vi "Demo.vi"() -> ()   [LabVIEW 2012, in "ProcessClass.lvclass"]
uses:
  ProcessClass.lvclass
panel:
  out "Process Names":string[](array[string])
  in  "停止":bool
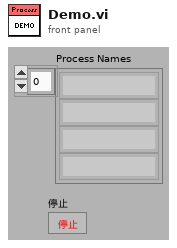
[diagram p1: front panel]
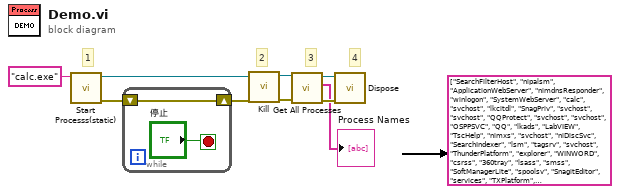
[diagram p0: block diagram]
diagram:
  (unwired) string[] ["SearchFilterHost", "nipalsm", "ApplicationWebServer", "nimdnsResponder", "winlogon", "SystemWebServer", "calc", "svchost", "lkcitdl", "SnagPriv", "svchost", "svchost", "QQProtect", "svchost", "svchost", "OSPPSVC", "QQ", "lkads", "LabVIEW", "TscHelp", "nimxs", "svchost", "niDiscSvc", "SearchIndexer", "lsm", "tagsrv", "svchost", "ThunderPlatform", "explorer", "WINWORD", "csrss", "360tray", "lsass", "smss", "SoftManagerLite", "spoolsv", "SnagitEditor", "services", "TXPlatform", "SearchProtocolHost", "csrss", "lktsrv", "svchost", "ZhuDongFangYu", "nidmsrv", "taskhost", "dwm", "Thunder", "PnkBstrA", "Snagit32", "wininit", "svchost", "System", "svchost", "svchost", "audiodg", "Idle"] ("Process Names")
  # "4"
  # "3"
  # "2"
  # "1"
  n1 = call "Start Processs(static).vi"("fileName"="calc.exe") -> ("error out"=w6:errorcluster, "ProcessClass 输出"=w4:refnum<class "ProcessClass.lvclass">)  [unwired: 9 in]
  n2 = while {
    shift-right: [w10] -> w5
    shift-left: w6 -> [w10]
    stop <- "停止" stop-if-true
  }
  n3 = call "Kill.vi"("error in (no error)"=w5, "ProcessClass 输入"=w4) -> ("error out"=w1:errorcluster, "ProcessClass 输出"=w7:refnum<class "ProcessClass.lvclass">)  [unwired: 8 in]
  n4 = call "Get All Processes.vi"("error in (no error)"=w1, "ProcessClass 输入"=w7) -> ("error out"=w8:errorcluster, "Process Names"=→"Process Names":string[], "ProcessClass 输出"=w9:refnum<class "ProcessClass.lvclass">)  [unwired: 7 in]
  n5 = call "Dispose.vi"("error in (no error)"=w8, "ProcessClass 输入"=w9) -> ()  [unwired: 8 in, 2 out]
